vi "subvi Robot Calculate Tile XY.vi"(1 "EProfileMove":bool, 2 "OverlapPriority":bool, 3 "MinOverlap":dbl, 4 "Magnification":u8, 5 "Objective":u8, 6 "Right":i32, 7 "Left":i32, 8 "Bottom":i32, 9 "Top":i32) -> (0 "TileInfo Cluster":T1)   [LabVIEW 2012]
panel:
  out "YOverlap":dbl
  out "XOverlap":dbl
  out "TileSuffix":string[](array[string])
  out "YTemp":i32[](array[numeric])
  out "XTemp":i32[](array[numeric])
  out "TileCoordinates":i32[][](array[numeric])
  out "YCoordinates":i32[](array[numeric])
  out "XCoordinates":i32[](array[numeric])
  out "FOVYLen":dbl
  out "FOVXLen":dbl
  out "TotalX":dbl
  out "TotalY":dbl
  out "YTiles":u16
  out "XTiles":u16
  out "PixelSize":dbl
  # "Output overlap\nin cluster is in %"
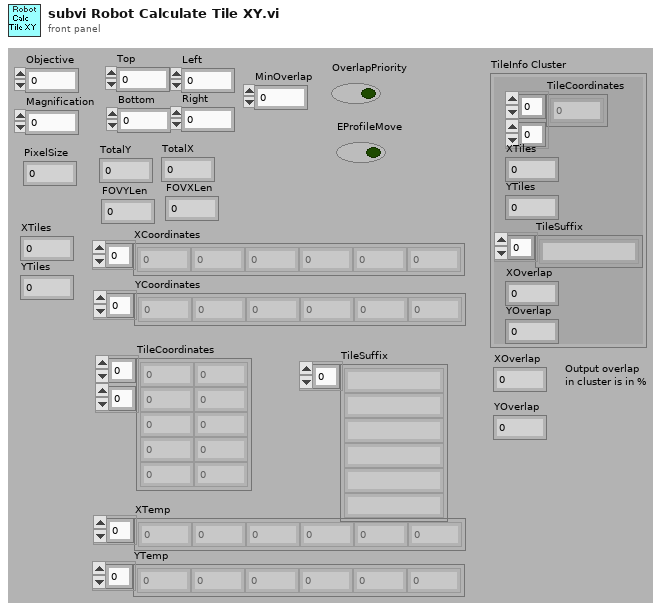
[diagram p1: front panel]
types:
  T1 = cluster{"TileCoordinates":i32[][], "XTiles":u16, "YTiles":u16, "TileSuffix":string[], "XOverlap":dbl, "YOverlap":dbl}
  T2 = cluster{"TileCoordinates":i32[][], "XTiles":u16, "YTiles":u16, "TileSuffix":string[], dbl, dbl}
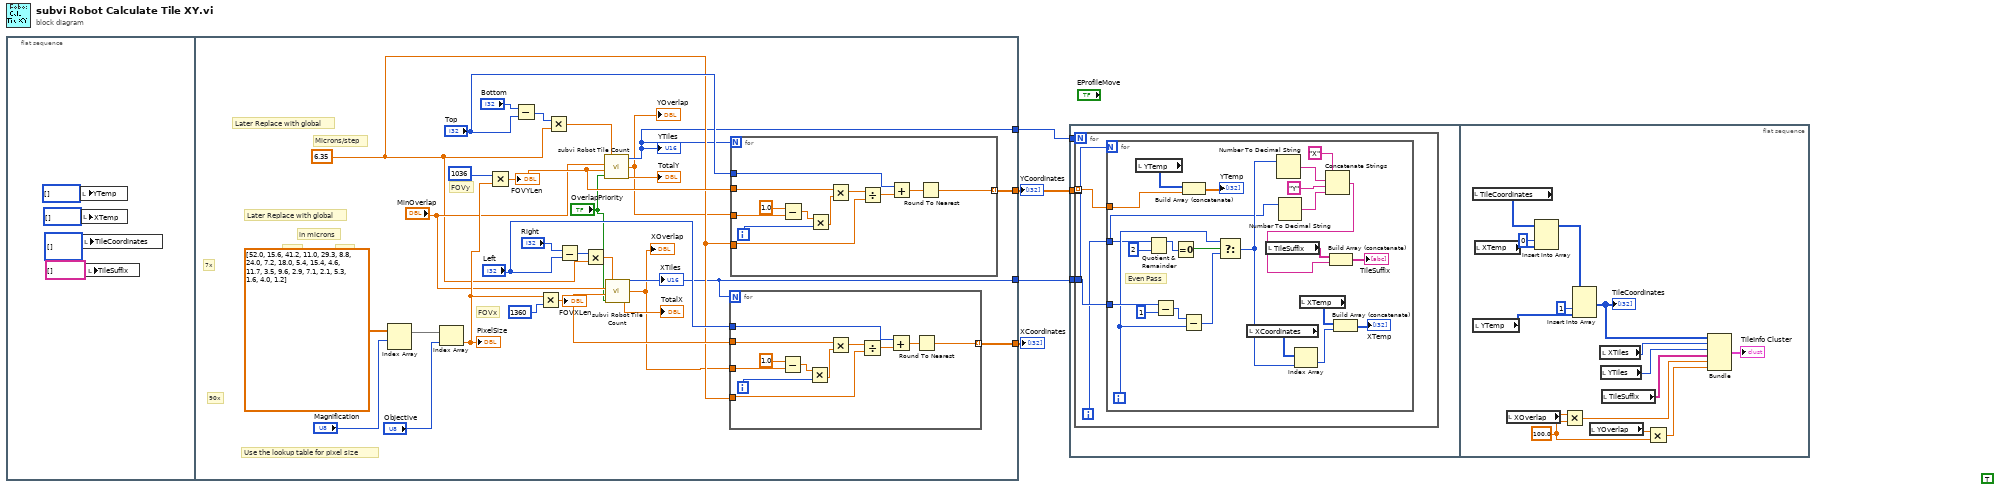
[diagram p0: block diagram]
diagram:
  (unwired) TRUE
  n1 = flat-sequence {
    tunnel: [w15] -> w1
    tunnel: [w14] -> w2
    tunnel: [w13] -> w4
    tunnel: [w12] -> w3
    frame #0 {
      n2 = local write "YTemp"(i32[] [] ("YTemp")) -> ()
      n3 = local write "XTemp"(i32[] [] ("XTemp")) -> ()
      n4 = local write "TileCoordinates"(i32[][] [] ("TileCoordinates")) -> ()
      n5 = local write "TileSuffix"(string[] [] ("TileSuffix")) -> ()
    }
    frame #1 {
      w16 = 6.35
      # "Later Replace with global"
      # "Later Replace with global"
      # "Microns/step"
      # "FOVy"
      # "FOVx"
      # "in microns"
      # "90x"
      # "7x"
      # "1.0X"
      # "0.3X"
      # "Use the lookup table for pixel size"
      n6 = Index Array(array=dbl[][] [[52.0, 15.6], [41.2, 11.0], [29.3, 8.8], [24.0, 7.2], [18.0, 5.4], [15.4, 4.6], [11.7, 3.5], [9.6, 2.9], [7.1, 2.1], [5.3, 1.6], [4.0, 1.2]], index (row)="Magnification") -> (element=w34:dbl[])  [unwired: 1 in]
      n7 = Index Array(array=w34, index="Objective") -> (element=w24:dbl)
      "PixelSize" <- w24
      n8 = Multiply(x=1036, y=w24) -> (x*y=w21:dbl)
      "FOVYLen" <- w21
      n9 = Subtract(x="Bottom", y="Top") -> (x-y=w31:i32)
      n10 = Multiply(x=w24, y=1360) -> (x*y=w18:dbl)
      "FOVXLen" <- w18
      n11 = Multiply(x=w31, y=w16) -> (x*y=w28:dbl)
      n12 = Subtract(x="Right", y="Left") -> (x-y=w27:i32)
      n13 = Multiply(x=w27, y=w16) -> (x*y=w23:dbl)
      n14 = call "subvi Robot Tile Count.vi"("OverlapPriority"="OverlapPriority", "TileLength"=w21, "MinOverlap"="MinOverlap", "MotorTravel"=w28) -> ("EdgelLength"=→"TotalY":dbl, "ActualOverlap"=w11:dbl, "NumTiles"=w15:u32)
      "YTiles" <- w15
      "YOverlap" <- w11
      n15 = call "subvi Robot Tile Count.vi"("OverlapPriority"="OverlapPriority", "TileLength"=w18, "MinOverlap"="MinOverlap", "MotorTravel"=w23) -> ("EdgelLength"=→"TotalX":dbl, "ActualOverlap"=w10:dbl, "NumTiles"=w14:u32)
      "XTiles" <- w14
      "XOverlap" <- w10
      n16 = for {
        N: w14 -> [_]
        tunnel: w10 -> [w48]
        tunnel: w18 -> [w43]
        tunnel: w16 -> [w42]
        tunnel: "Left" -> [w39]
        tunnel: [w37] -> w12 mode=indexing
        i -> [w45]
        n17 = Subtract(x=1.0, y=w48) -> (x-y=w46:dbl)
        n18 = Multiply(x=w46, y=w45) -> (x*y=w44:dbl)
        n19 = Multiply(x=w43, y=w44) -> (x*y=w41:dbl)
        n20 = Divide(x=w41, y=w42) -> (x/y=w40:dbl)
        n21 = Add(x=w39, y=w40) -> (x+y=w38:dbl)
        n22 = Round To Nearest(number=w38) -> (nearest integer value=w37:dbl)
      }
      n23 = for {
        N: w15 -> [_]
        tunnel: w11 -> [w60]
        tunnel: w21 -> [w55]
        tunnel: w16 -> [w54]
        tunnel: "Top" -> [w51]
        tunnel: [w49] -> w13 mode=indexing
        i -> [w57]
        n24 = Subtract(x=1.0, y=w60) -> (x-y=w58:dbl)
        n25 = Multiply(x=w58, y=w57) -> (x*y=w56:dbl)
        n26 = Multiply(x=w55, y=w56) -> (x*y=w53:dbl)
        n27 = Divide(x=w53, y=w54) -> (x/y=w52:dbl)
        n28 = Add(x=w51, y=w52) -> (x+y=w50:dbl)
        n29 = Round To Nearest(number=w50) -> (nearest integer value=w49:dbl)
      }
    }
  }
  n30 = flat-sequence {
    tunnel: w1 -> [w63]
    tunnel: w2 -> [w62]
    tunnel: w4 -> [w61]
    frame #0 {
      n31 = for {
        N: w63 -> [_]
        tunnel: w62 -> [w65]
        tunnel: w61 -> [_] mode=indexing
        tunnel: w61 -> [w66] mode=indexing
        i -> [w64]
        n32 = for {
          N: w65 -> [_]
          tunnel: w66 -> [w86]
          tunnel: w65 -> [w85]
          tunnel: w64 -> [w74]
          i -> [w83]
          # "Even Pass"
          n33 = local read "YTemp"() -> (w88:i32[])
          n34 = Quotient & Remainder(x=w74, y=2) -> (x-y*floor(x/y)=w76:i32)  [unwired: 1 out]
          n35 = Subtract(x=w85, y=u32 1) -> (x-y=w82:u32)
          n36 = Equal To 0?(x=w76) -> (x = 0?=w89:bool)
          n37 = Subtract(x=w82, y=w83) -> (x-y=w81:u32)
          n38 = Build Array (concatenate)(w88, w86) -> (→"YTemp":dbl[])
          n39 = Select(t=w83, s=w89, f=w81) -> (s? t:f=w75:u32)
          n40 = local read "XCoordinates"() -> (w78:i32[])
          n41 = local read "TileSuffix"() -> (w72:string[])
          n42 = Number To Decimal String(number=w75) -> (decimal integer string=w73:string)  [unwired: 1 out]
          n43 = Number To Decimal String(number=w74) -> (decimal integer string=w69:string)  [unwired: 1 out]
          n44 = Index Array(array=w78, index=w75) -> (element=w77:i32)
          n45 = local read "XTemp"() -> (w80:i32[])
          n46 = Concatenate Strings("X" ("string"), w73, "Y" ("string"), w69) -> (w70:string)
          n47 = Build Array (concatenate)(w72, w70) -> (→"TileSuffix":string[])
          n48 = Build Array (concatenate)(w80, w77) -> (→"XTemp":i32[])
        }
      }
    }
    frame #1 {
      w92 = 100.0 ("y")
      n49 = local read "TileCoordinates"() -> (w106:i32[][])
      n50 = local read "YTemp"() -> (w102:i32[])
      n51 = local read "XTemp"() -> (w105:i32[])
      n52 = local read "XOverlap"() -> (w95:dbl)
      n53 = Insert Into Array(array=w106, index (col)=0 ("disabled index (col)"), new element=w105) -> (w103:i32[][])  [unwired: 1 in]
      n54 = Multiply(x=w95, y=w92) -> (x*y=w94:dbl)
      n55 = Insert Into Array(array=w103, index (col)=1 ("disabled index (col)"), new element=w102) -> (w100:i32[][])  [unwired: 1 in]
      "TileCoordinates" <- w100
      n56 = local read "YOverlap"() -> (w93:dbl)
      n57 = local read "XTiles"() -> (w97:u16)
      n58 = local read "YTiles"() -> (w98:u16)
      n59 = local read "TileSuffix"() -> (w99:string[])
      n60 = Multiply(x=w93, y=w92) -> (x*y=w91:dbl)
      n61 = Bundle("TileCoordinates"=w100, "XTiles"=w97, "YTiles"=w98, "TileSuffix"=w99, w94, w91) -> (→"TileInfo Cluster":T2)  [unwired: 1 out]
    }
  }
  "XCoordinates" <- w3
  "YCoordinates" <- w4
